vi "Test Single Gas Calibration.vi"() -> ()   [LabVIEW 2015]
uses:
  Filter Result.ctl
  Controls/Test Config.ctl
  Controls/Gas Mixture.ctl
  CAN Communication/PAS/Typedefs/ADC Gains.ctl
  Controls/Filter Sequence.ctl
  Controls/Functional Test.ctl
  CAN Communication/PAS/PAS.lvclass
panel:
  out "length":i32
  out "F-format string":string
  in  "Test Config":T1={"Chopper RPM"=140, "IR Power"=5, "Conc Tolerance"=0.0, "Gas Stable Time"=0, "A-D Settle"=0, "Samples"=0, "Filter Time"=0, "Gas Mixtures"=[], "Filter Sequences"=[{"Filter"=1, "Phase"=60.0}, {"Filter"=2, "Phase"=60.0}, {"Filter"=3, "Phase"=60.0}, {"Filter"=4, "Phase"=60.0}, {"Filter"=5, "Phase"=60.0}, {"Filter"=6, "Phase"=60.0}, {"Filter"=7, "Phase"=55.0}, {"Filter"=8, "Phase"=55.0}, {"Filter"=9, "Phase"=50.0}], "Functional Test"={"Mic Test ON ADC Max"=0.0, "Mic Test ON ADC Min"=0.0, "Mic Test OFF ADC Max"=0.0, "Mic Test OFF ADC Min"=0.0, "Mic Test IC ADC Max"=0.0, "Mic Test IC ADC Min"=0.0, "IR Emitter ON ADC Max"=0.0, "IR Emitter ON ADC Min"=0.0, "IR Emitter OFF ADC Max"=0.0, "IR Emitter OFF ADC Min"=0.0}, "Initial Flow Rate"=0.0, "Max Flow Rate"=0.0} {"Gas Mixtures"."ADC Gains" items=["0"=0, "3"=3, "4"=4, "5"=5, "6"=6, "7"=7]; "Conc Tolerance" min=0.0 max=100.0 step=1.0; "IR Power" min=2 max=5 step=1; "Chopper RPM" min=140 max=1000 step=1}
  out "Filter Results":T6[](array[typedef])
  out "error out":errorcluster
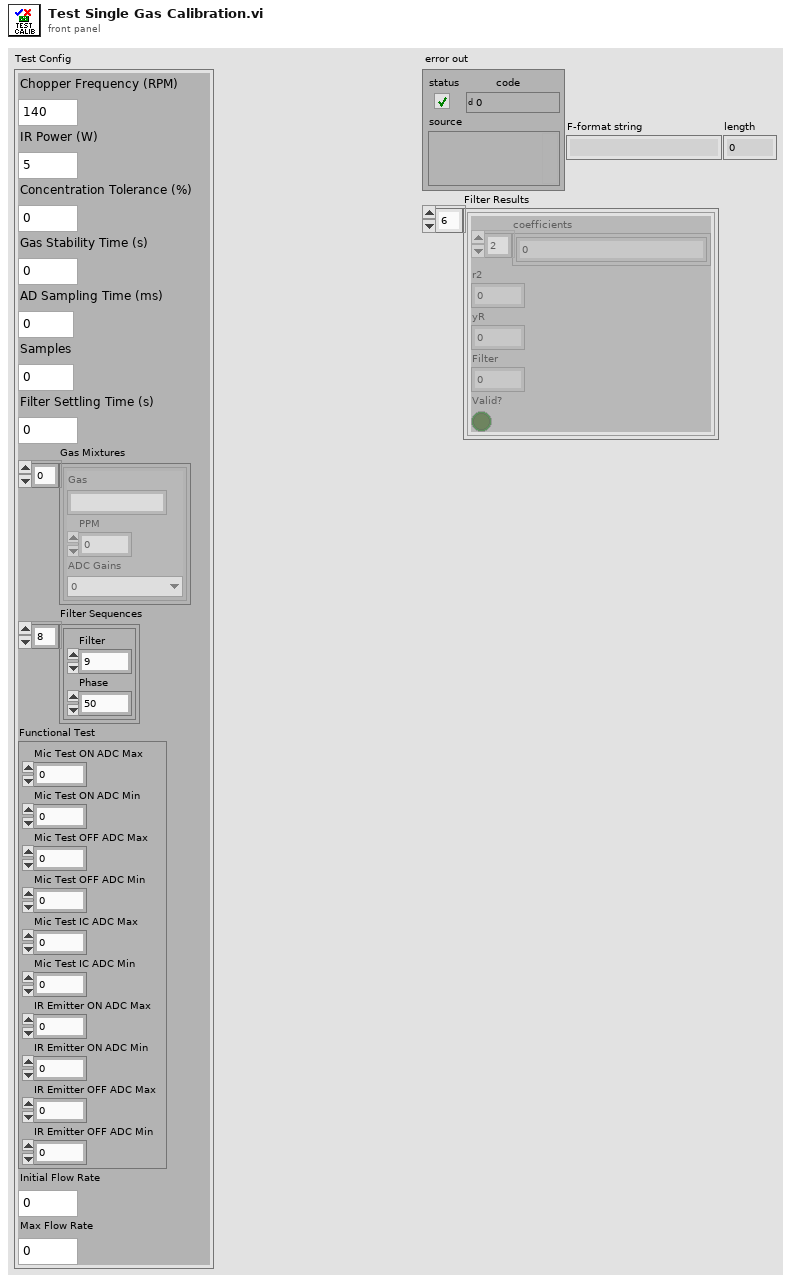
[diagram p1: front panel]
types:
  T1 = typedef "Test Config.ctl" = cluster{"Chopper RPM":u16, "IR Power":u8, "Conc Tolerance":dbl, "Gas Stable Time":u16, "A-D Settle":u16, "Samples":u16, "Filter Time":u16, "Gas Mixtures":T2[], "Filter Sequences":T4[], "Functional Test":T5, "Initial Flow Rate":sgl, "Max Flow Rate":sgl}
  T2 = typedef "Gas Mixture.ctl" = cluster{"Gas":string, "PPM":dbl, "ADC Gains":T3}
  T3 = typedef "PAS.lvclass/ADC Gains.ctl" = u16
  T4 = typedef "Filter Sequence.ctl" = cluster{"Filter":u8, "Phase":dbl}
  T5 = typedef "Functional Test.ctl" = cluster{"Mic Test ON ADC Max":dbl, "Mic Test ON ADC Min":dbl, "Mic Test OFF ADC Max":dbl, "Mic Test OFF ADC Min":dbl, "Mic Test IC ADC Max":dbl, "Mic Test IC ADC Min":dbl, "IR Emitter ON ADC Max":dbl, "IR Emitter ON ADC Min":dbl, "IR Emitter OFF ADC Max":dbl, "IR Emitter OFF ADC Min":dbl}
  T6 = typedef "Filter Result.ctl" = cluster{"coefficients":dbl[], "r2":dbl, "yR":dbl, "Filter":i32, "Valid?":bool}
  T7 = typedef "Test Info.ctl" = cluster{"Gas Counter":u16, "Filter Counter":u16, "ADC Samples":dbl[], "Gas Timeout":u16, "Notes":string, "Moisture":dbl, "PPM":dbl, "Mean":dbl, "STD":dbl, "Gas":string, "Temp":dbl, "Pressure":dbl, "Filter":u8, "Phase":dbl, "numSamples":u8}
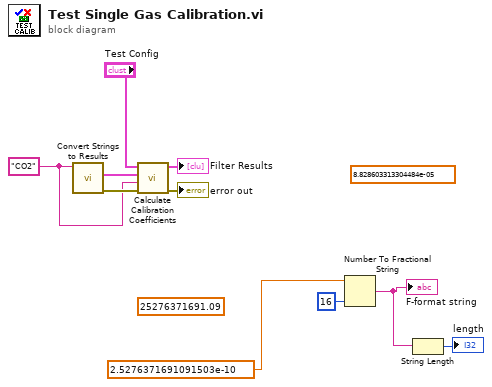
[diagram p0: block diagram]
diagram:
  (unwired) 25276371691.09
  (unwired) sgl 8.828603e-05
  w7 = "CO2" ("Gas")
  n1 = call "Convert Strings to Results.vi"("Gas"=w7) -> ("error out"=w10:errorcluster, "Results"=w9:T7[])  [unwired: 9 in]
  n2 = call "Calculate Calibration Coefficients.vi"("error in (no error)"=w10, "Gas"=w7, "Results"=w9, "Test Config"="Test Config") -> ("error out"=→"error out":errorcluster, "Filter Results"=→"Filter Results":T6[])  [unwired: 6 in]
  n3 = Number To Fractional String(number=2.5276371691091503e-10, precision (6)=i16 16) -> (F-format string=w3:string)  [unwired: 2 in]
  "F-format string" <- w3
  n4 = String Length(string=w3) -> (length=→"length":i32)
